vi "find strasse.vi"(11 "Karte in":T1={"Kreuzungen"=[{"Name"="A1", "Identifikation"=0, "Koord"={"x"=100.0, "y"=100.0}, "Anzahl Abgänge"=1}, {"Name"="A2", "Identifikation"=1, "Koord"={"x"=180.0, "y"=180.0}, "Anzahl Abgänge"=1}, {"Name"="A3", "Identifikation"=2, "Koord"={"x"=210.0, "y"=210.0}, "Anzahl Abgänge"=3}, {"Name"="A4", "Identifikation"=3, "Koord"={"x"=300.0, "y"=300.0}, "Anzahl Abgänge"=3}, {"Name"="A5", "Identifikation"=4, "Koord"={"x"=320.0, "y"=320.0}, "Anzahl Abgänge"=1}, {"Name"="A6", "Identifikation"=5, "Koord"={"x"=40.0, "y"=40.0}, "Anzahl Abgänge"=1}, {"Name"="A7", "Identifikation"=6, "Koord"={"x"=90.0, "y"=90.0}, "Anzahl Abgänge"=3}, {"Name"="A8", "Identifikation"=7, "Koord"={"x"=100.0, "y"=100.0}, "Anzahl Abgänge"=2}, {"Name"="A9", "Identifikation"=8, "Koord"={"x"=90.0, "y"=90.0}, "Anzahl Abgänge"=3}, {"Name"="A10", "Identifikation"=9, "Koord"={"x"=180.0, "y"=180.0}, "Anzahl Abgänge"=3}, {"Name"="A11", "Identifikation"=10, "Koord"={"x"=210.0, "y"=210.0}, "Anzahl Abgänge"=3}, {"Name"="A12", "Identifikation"=11, "Koord"={"x"=180.0, "y"=180.0}, "Anzahl Abgänge"=3}, {"Name"="A13", "Identifikation"=12, "Koord"={"x"=210.0, "y"=210.0}, "Anzahl Abgänge"=3}, {"Name"="A14", "Identifikation"=13, "Koord"={"x"=270.0, "y"=270.0}, "Anzahl Abgänge"=3}, {"Name"="A15", "Identifikation"=14, "Koord"={"x"=300.0, "y"=300.0}, "Anzahl Abgänge"=1}, {"Name"="A16", "Identifikation"=15, "Koord"={"x"=270.0, "y"=270.0}, "Anzahl Abgänge"=3}, {"Name"="A17", "Identifikation"=16, "Koord"={"x"=340.0, "y"=340.0}, "Anzahl Abgänge"=1}, {"Name"="A18", "Identifikation"=17, "Koord"={"x"=180.0, "y"=180.0}, "Anzahl Abgänge"=1}, {"Name"="A19", "Identifikation"=18, "Koord"={"x"=90.0, "y"=90.0}, "Anzahl Abgänge"=1}, {"Name"="A20", "Identifikation"=19, "Koord"={"x"=60.0, "y"=60.0}, "Anzahl Abgänge"=2}, {"Name"="A21", "Identifikation"=20, "Koord"={"x"=160.0, "y"=160.0}, "Anzahl Abgänge"=2}, {"Name"="A22", "Identifikation"=21, "Koord"={"x"=60.0, "y"=60.0}, "Anzahl Abgänge"=1}, {"Name"="A23", "Identifikation"=22, "Koord"={"x"=160.0, "y"=160.0}, "Anzahl Abgänge"=2}, {"Name"="A24", "Identifikation"=23, "Koord"={"x"=270.0, "y"=270.0}, "Anzahl Abgänge"=3}, {"Name"="A25", "Identifikation"=24, "Koord"={"x"=340.0, "y"=340.0}, "Anzahl Abgänge"=1}], "Strassen"=[{"Name"="A 1 8", "Identifikation"=0, "Verbindungen"=[{"Start_Kr"=0, "Ziel_Kr"=7}, {"Start_Kr"=7, "Ziel_Kr"=0}], "Breite"=40, "Strassen_Typ"=enum."Stadt"}, {"Name"="A 2 3", "Identifikation"=1, "Verbindungen"=[{"Start_Kr"=1, "Ziel_Kr"=2}, {"Start_Kr"=2, "Ziel_Kr"=1}], "Breite"=40, "Strassen_Typ"=enum."Innenstadt"}, {"Name"="A 3 4", "Identifikation"=2, "Verbindungen"=[{"Start_Kr"=2, "Ziel_Kr"=3}, {"Start_Kr"=3, "Ziel_Kr"=2}], "Breite"=40, "Strassen_Typ"=enum."Innenstadt"}, {"Name"="A 311", "Identifikation"=3, "Verbindungen"=[{"Start_Kr"=2, "Ziel_Kr"=10}, {"Start_Kr"=10, "Ziel_Kr"=2}], "Breite"=40, "Strassen_Typ"=enum."Innenstadt"}, {"Name"="A 4 5", "Identifikation"=4, "Verbindungen"=[{"Start_Kr"=3, "Ziel_Kr"=4}, {"Start_Kr"=4, "Ziel_Kr"=3}], "Breite"=40, "Strassen_Typ"=enum."Innenstadt"}, {"Name"="A 6 7", "Identifikation"=5, "Verbindungen"=[{"Start_Kr"=5, "Ziel_Kr"=6}, {"Start_Kr"=6, "Ziel_Kr"=5}], "Breite"=40, "Strassen_Typ"=enum."Stadt"}, {"Name"="A 7 8", "Identifikation"=6, "Verbindungen"=[{"Start_Kr"=6, "Ziel_Kr"=7}, {"Start_Kr"=7, "Ziel_Kr"=6}], "Breite"=40, "Strassen_Typ"=enum."Stadt"}, {"Name"="A 7 9", "Identifikation"=7, "Verbindungen"=[{"Start_Kr"=6, "Ziel_Kr"=8}, {"Start_Kr"=8, "Ziel_Kr"=6}], "Breite"=40, "Strassen_Typ"=enum."Stadt"}, {"Name"="A 910", "Identifikation"=8, "Verbindungen"=[{"Start_Kr"=8, "Ziel_Kr"=9}, {"Start_Kr"=9, "Ziel_Kr"=8}], "Breite"=40, "Strassen_Typ"=enum."Innenstadt"}, {"Name"="A 919", "Identifikation"=9, "Verbindungen"=[{"Start_Kr"=8, "Ziel_Kr"=18}, {"Start_Kr"=18, "Ziel_Kr"=8}], "Breite"=40, "Strassen_Typ"=enum."Stadt"}, {"Name"="A1011", "Identifikation"=10, "Verbindungen"=[{"Start_Kr"=9, "Ziel_Kr"=10}, {"Start_Kr"=10, "Ziel_Kr"=9}], "Breite"=40, "Strassen_Typ"=enum."Innenstadt"}, {"Name"="A1012", "Identifikation"=11, "Verbindungen"=[{"Start_Kr"=9, "Ziel_Kr"=11}, {"Start_Kr"=11, "Ziel_Kr"=9}], "Breite"=40, "Strassen_Typ"=enum."Innenstadt"}, {"Name"="A1113", "Identifikation"=12, "Verbindungen"=[{"Start_Kr"=10, "Ziel_Kr"=12}, {"Start_Kr"=12, "Ziel_Kr"=10}], "Breite"=40, "Strassen_Typ"=enum."Innenstadt"}, {"Name"="A1213", "Identifikation"=13, "Verbindungen"=[{"Start_Kr"=11, "Ziel_Kr"=12}, {"Start_Kr"=12, "Ziel_Kr"=11}], "Breite"=40, "Strassen_Typ"=enum."Innenstadt"}, {"Name"="A1218", "Identifikation"=14, "Verbindungen"=[{"Start_Kr"=11, "Ziel_Kr"=17}, {"Start_Kr"=17, "Ziel_Kr"=11}], "Breite"=40, "Strassen_Typ"=enum."Innenstadt"}, {"Name"="A1314", "Identifikation"=15, "Verbindungen"=[{"Start_Kr"=12, "Ziel_Kr"=13}, {"Start_Kr"=13, "Ziel_Kr"=12}], "Breite"=40, "Strassen_Typ"=enum."Innenstadt"}, {"Name"="A1415", "Identifikation"=16, "Verbindungen"=[{"Start_Kr"=13, "Ziel_Kr"=14}, {"Start_Kr"=14, "Ziel_Kr"=13}], "Breite"=40, "Strassen_Typ"=enum."Innenstadt"}, {"Name"="A1416", "Identifikation"=17, "Verbindungen"=[{"Start_Kr"=13, "Ziel_Kr"=15}, {"Start_Kr"=15, "Ziel_Kr"=13}], "Breite"=40, "Strassen_Typ"=enum."Innenstadt"}, {"Name"="A 415", "Identifikation"=18, "Verbindungen"=[{"Start_Kr"=14, "Ziel_Kr"=3}], "Breite"=40, "Strassen_Typ"=enum."Innenstadt"}, {"Name"="A1617", "Identifikation"=19, "Verbindungen"=[{"Start_Kr"=15, "Ziel_Kr"=16}, {"Start_Kr"=16, "Ziel_Kr"=15}], "Breite"=40, "Strassen_Typ"=enum."Stadt"}, {"Name"="A1624", "Identifikation"=20, "Verbindungen"=[{"Start_Kr"=15, "Ziel_Kr"=23}, {"Start_Kr"=23, "Ziel_Kr"=15}], "Breite"=40, "Strassen_Typ"=enum."Stadt"}, {"Name"="A2021", "Identifikation"=21, "Verbindungen"=[{"Start_Kr"=19, "Ziel_Kr"=20}, {"Start_Kr"=20, "Ziel_Kr"=19}], "Breite"=40, "Strassen_Typ"=enum."Land"}, {"Name"="A2022", "Identifikation"=22, "Verbindungen"=[{"Start_Kr"=19, "Ziel_Kr"=21}, {"Start_Kr"=21, "Ziel_Kr"=19}], "Breite"=40, "Strassen_Typ"=enum."Land"}, {"Name"="A2123", "Identifikation"=23, "Verbindungen"=[{"Start_Kr"=20, "Ziel_Kr"=22}, {"Start_Kr"=22, "Ziel_Kr"=20}], "Breite"=40, "Strassen_Typ"=enum."Land"}, {"Name"="A2324", "Identifikation"=24, "Verbindungen"=[{"Start_Kr"=22, "Ziel_Kr"=23}, {"Start_Kr"=23, "Ziel_Kr"=22}], "Breite"=40, "Strassen_Typ"=enum."Land"}, {"Name"="A2425", "Identifikation"=25, "Verbindungen"=[{"Start_Kr"=23, "Ziel_Kr"=24}, {"Start_Kr"=24, "Ziel_Kr"=23}], "Breite"=40, "Strassen_Typ"=enum."Land"}], "Häuser"=[{"Name"="Haus1", "Hausnummer"=0, "Polygon"=[{"x"=220.0, "y"=40.0}, {"x"=280.0, "y"=40.0}, {"x"=280.0, "y"=0.0}, {"x"=220.0, "y"=0.0}, {"x"=250.0, "y"=20.0}], "Strassennummer"=0, "Türe"={"x"=250.0, "y"=40.0}}, {"Name"="Haus2", "Hausnummer"=1, "Polygon"=[{"x"=280.0, "y"=40.0}, {"x"=340.0, "y"=40.0}, {"x"=340.0, "y"=0.0}, {"x"=280.0, "y"=0.0}, {"x"=310.0, "y"=20.0}], "Strassennummer"=0, "Türe"={"x"=310.0, "y"=40.0}}, {"Name"="Haus3", "Hausnummer"=2, "Polygon"=[{"x"=20.0, "y"=60.0}, {"x"=80.0, "y"=60.0}, {"x"=80.0, "y"=20.0}, {"x"=20.0, "y"=20.0}, {"x"=50.0, "y"=40.0}], "Strassennummer"=0, "Türe"={"x"=50.0, "y"=60.0}}, {"Name"="Haus4", "Hausnummer"=3, "Polygon"=[{"x"=120.0, "y"=40.0}, {"x"=120.0, "y"=100.0}, {"x"=160.0, "y"=100.0}, {"x"=160.0, "y"=40.0}, {"x"=140.0, "y"=70.0}], "Strassennummer"=0, "Türe"={"x"=120.0, "y"=70.0}}, {"Name"="Haus5", "Hausnummer"=4, "Polygon"=[{"x"=340.0, "y"=40.0}, {"x"=340.0, "y"=100.0}, {"x"=380.0, "y"=100.0}, {"x"=380.0, "y"=40.0}, {"x"=360.0, "y"=70.0}], "Strassennummer"=0, "Türe"={"x"=340.0, "y"=70.0}}, {"Name"="Haus6", "Hausnummer"=5, "Polygon"=[{"x"=20.0, "y"=120.0}, {"x"=20.0, "y"=180.0}, {"x"=60.0, "y"=180.0}, {"x"=60.0, "y"=120.0}, {"x"=40.0, "y"=150.0}], "Strassennummer"=0, "Türe"={"x"=40.0, "y"=120.0}}, {"Name"="Haus7", "Hausnummer"=6, "Polygon"=[{"x"=180.0, "y"=100.0}, {"x"=120.0, "y"=100.0}, {"x"=120.0, "y"=140.0}, {"x"=180.0, "y"=140.0}, {"x"=150.0, "y"=120.0}], "Strassennummer"=0, "Türe"={"x"=180.0, "y"=120.0}}, {"Name"="Haus8", "Hausnummer"=7, "Polygon"=[{"x"=320.0, "y"=140.0}, {"x"=380.0, "y"=140.0}, {"x"=380.0, "y"=100.0}, {"x"=320.0, "y"=100.0}, {"x"=350.0, "y"=120.0}], "Strassennummer"=0, "Türe"={"x"=320.0, "y"=120.0}}, {"Name"="Haus9", "Hausnummer"=8, "Polygon"=[{"x"=240.0, "y"=100.0}, {"x"=240.0, "y"=160.0}, {"x"=280.0, "y"=160.0}, {"x"=280.0, "y"=100.0}, {"x"=260.0, "y"=130.0}], "Strassennummer"=0, "Türe"={"x"=240.0, "y"=130.0}}, {"Name"="Haus10", "Hausnummer"=9, "Polygon"=[{"x"=320.0, "y"=140.0}, {"x"=320.0, "y"=200.0}, {"x"=360.0, "y"=200.0}, {"x"=360.0, "y"=140.0}, {"x"=340.0, "y"=170.0}], "Strassennummer"=0, "Türe"={"x"=320.0, "y"=170.0}}, {"Name"="Haus11", "Hausnummer"=10, "Polygon"=[{"x"=45.0, "y"=240.0}, {"x"=45.0, "y"=180.0}, {"x"=5.0, "y"=180.0}, {"x"=5.0, "y"=240.0}, {"x"=25.0, "y"=210.0}], "Strassennummer"=0, "Türe"={"x"=45.0, "y"=210.0}}, {"Name"="Haus12", "Hausnummer"=11, "Polygon"=[{"x"=200.0, "y"=220.0}, {"x"=200.0, "y"=280.0}, {"x"=240.0, "y"=280.0}, {"x"=240.0, "y"=220.0}, {"x"=220.0, "y"=250.0}], "Strassennummer"=0, "Türe"={"x"=220.0, "y"=220.0}}, {"Name"="Haus13", "Hausnummer"=12, "Polygon"=[{"x"=160.0, "y"=260.0}, {"x"=160.0, "y"=200.0}, {"x"=120.0, "y"=200.0}, {"x"=120.0, "y"=260.0}, {"x"=140.0, "y"=230.0}], "Strassennummer"=0, "Türe"={"x"=160.0, "y"=230.0}}, {"Name"="Haus14", "Hausnummer"=13, "Polygon"=[{"x"=60.0, "y"=240.0}, {"x"=0.0, "y"=240.0}, {"x"=0.0, "y"=280.0}, {"x"=60.0, "y"=280.0}, {"x"=30.0, "y"=260.0}], "Strassennummer"=0, "Türe"={"x"=60.0, "y"=260.0}}, {"Name"="Haus15", "Hausnummer"=14, "Polygon"=[{"x"=360.0, "y"=280.0}, {"x"=300.0, "y"=280.0}, {"x"=300.0, "y"=320.0}, {"x"=360.0, "y"=320.0}, {"x"=330.0, "y"=300.0}], "Strassennummer"=0, "Türe"={"x"=330.0, "y"=280.0}}, {"Name"="Haus16", "Hausnummer"=15, "Polygon"=[{"x"=130.0, "y"=300.0}, {"x"=190.0, "y"=300.0}, {"x"=190.0, "y"=260.0}, {"x"=130.0, "y"=260.0}, {"x"=160.0, "y"=280.0}], "Strassennummer"=0, "Türe"={"x"=160.0, "y"=300.0}}, {"Name"="Haus17", "Hausnummer"=16, "Polygon"=[{"x"=240.0, "y"=350.0}, {"x"=240.0, "y"=290.0}, {"x"=200.0, "y"=290.0}, {"x"=200.0, "y"=350.0}, {"x"=220.0, "y"=320.0}], "Strassennummer"=0, "Türe"={"x"=240.0, "y"=320.0}}, {"Name"="Haus18", "Hausnummer"=17, "Polygon"=[{"x"=300.0, "y"=360.0}, {"x"=360.0, "y"=360.0}, {"x"=360.0, "y"=320.0}, {"x"=300.0, "y"=320.0}, {"x"=330.0, "y"=340.0}], "Strassennummer"=0, "Türe"={"x"=330.0, "y"=360.0}}, {"Name"="Haus19", "Hausnummer"=18, "Polygon"=[{"x"=90.0, "y"=400.0}, {"x"=30.0, "y"=400.0}, {"x"=30.0, "y"=440.0}, {"x"=90.0, "y"=440.0}, {"x"=60.0, "y"=420.0}], "Strassennummer"=0, "Türe"={"x"=60.0, "y"=400.0}}, {"Name"="Poststelle", "Hausnummer"=19, "Polygon"=[{"x"=160.0, "y"=40.0}, {"x"=220.0, "y"=40.0}, {"x"=220.0, "y"=0.0}, {"x"=160.0, "y"=0.0}, {"x"=190.0, "y"=20.0}], "Strassennummer"=0, "Türe"={"x"=190.0, "y"=40.0}}]}) -> (3 "Karte out":T1={"Kreuzungen"=[{"Name"="A1", "Identifikation"=0, "Koord"={"x"=100.0, "y"=100.0}, "Anzahl Abgänge"=1}, {"Name"="A2", "Identifikation"=1, "Koord"={"x"=180.0, "y"=180.0}, "Anzahl Abgänge"=1}, {"Name"="A3", "Identifikation"=2, "Koord"={"x"=210.0, "y"=210.0}, "Anzahl Abgänge"=3}, {"Name"="A4", "Identifikation"=3, "Koord"={"x"=300.0, "y"=300.0}, "Anzahl Abgänge"=3}, {"Name"="A5", "Identifikation"=4, "Koord"={"x"=320.0, "y"=320.0}, "Anzahl Abgänge"=1}, {"Name"="A6", "Identifikation"=5, "Koord"={"x"=40.0, "y"=40.0}, "Anzahl Abgänge"=1}, {"Name"="A7", "Identifikation"=6, "Koord"={"x"=90.0, "y"=90.0}, "Anzahl Abgänge"=3}, {"Name"="A8", "Identifikation"=7, "Koord"={"x"=100.0, "y"=100.0}, "Anzahl Abgänge"=2}, {"Name"="A9", "Identifikation"=8, "Koord"={"x"=90.0, "y"=90.0}, "Anzahl Abgänge"=3}, {"Name"="A10", "Identifikation"=9, "Koord"={"x"=180.0, "y"=180.0}, "Anzahl Abgänge"=3}, {"Name"="A11", "Identifikation"=10, "Koord"={"x"=210.0, "y"=210.0}, "Anzahl Abgänge"=3}, {"Name"="A12", "Identifikation"=11, "Koord"={"x"=180.0, "y"=180.0}, "Anzahl Abgänge"=3}, {"Name"="A13", "Identifikation"=12, "Koord"={"x"=210.0, "y"=210.0}, "Anzahl Abgänge"=3}, {"Name"="A14", "Identifikation"=13, "Koord"={"x"=270.0, "y"=270.0}, "Anzahl Abgänge"=3}, {"Name"="A15", "Identifikation"=14, "Koord"={"x"=300.0, "y"=300.0}, "Anzahl Abgänge"=1}, {"Name"="A16", "Identifikation"=15, "Koord"={"x"=270.0, "y"=270.0}, "Anzahl Abgänge"=3}, {"Name"="A17", "Identifikation"=16, "Koord"={"x"=340.0, "y"=340.0}, "Anzahl Abgänge"=1}, {"Name"="A18", "Identifikation"=17, "Koord"={"x"=180.0, "y"=180.0}, "Anzahl Abgänge"=1}, {"Name"="A19", "Identifikation"=18, "Koord"={"x"=90.0, "y"=90.0}, "Anzahl Abgänge"=1}, {"Name"="A20", "Identifikation"=19, "Koord"={"x"=60.0, "y"=60.0}, "Anzahl Abgänge"=2}, {"Name"="A21", "Identifikation"=20, "Koord"={"x"=160.0, "y"=160.0}, "Anzahl Abgänge"=2}, {"Name"="A22", "Identifikation"=21, "Koord"={"x"=60.0, "y"=60.0}, "Anzahl Abgänge"=1}, {"Name"="A23", "Identifikation"=22, "Koord"={"x"=160.0, "y"=160.0}, "Anzahl Abgänge"=2}, {"Name"="A24", "Identifikation"=23, "Koord"={"x"=270.0, "y"=270.0}, "Anzahl Abgänge"=3}, {"Name"="A25", "Identifikation"=24, "Koord"={"x"=340.0, "y"=340.0}, "Anzahl Abgänge"=1}], "Strassen"=[{"Name"="A 1 8", "Identifikation"=0, "Verbindungen"=[{"Start_Kr"=0, "Ziel_Kr"=7}, {"Start_Kr"=7, "Ziel_Kr"=0}], "Breite"=40, "Strassen_Typ"=enum."Stadt"}, {"Name"="A 2 3", "Identifikation"=1, "Verbindungen"=[{"Start_Kr"=1, "Ziel_Kr"=2}, {"Start_Kr"=2, "Ziel_Kr"=1}], "Breite"=40, "Strassen_Typ"=enum."Innenstadt"}, {"Name"="A 3 4", "Identifikation"=2, "Verbindungen"=[{"Start_Kr"=2, "Ziel_Kr"=3}, {"Start_Kr"=3, "Ziel_Kr"=2}], "Breite"=40, "Strassen_Typ"=enum."Innenstadt"}, {"Name"="A 311", "Identifikation"=3, "Verbindungen"=[{"Start_Kr"=2, "Ziel_Kr"=10}, {"Start_Kr"=10, "Ziel_Kr"=2}], "Breite"=40, "Strassen_Typ"=enum."Innenstadt"}, {"Name"="A 4 5", "Identifikation"=4, "Verbindungen"=[{"Start_Kr"=3, "Ziel_Kr"=4}, {"Start_Kr"=4, "Ziel_Kr"=3}], "Breite"=40, "Strassen_Typ"=enum."Innenstadt"}, {"Name"="A 6 7", "Identifikation"=5, "Verbindungen"=[{"Start_Kr"=5, "Ziel_Kr"=6}, {"Start_Kr"=6, "Ziel_Kr"=5}], "Breite"=40, "Strassen_Typ"=enum."Stadt"}, {"Name"="A 7 8", "Identifikation"=6, "Verbindungen"=[{"Start_Kr"=6, "Ziel_Kr"=7}, {"Start_Kr"=7, "Ziel_Kr"=6}], "Breite"=40, "Strassen_Typ"=enum."Stadt"}, {"Name"="A 7 9", "Identifikation"=7, "Verbindungen"=[{"Start_Kr"=6, "Ziel_Kr"=8}, {"Start_Kr"=8, "Ziel_Kr"=6}], "Breite"=40, "Strassen_Typ"=enum."Stadt"}, {"Name"="A 910", "Identifikation"=8, "Verbindungen"=[{"Start_Kr"=8, "Ziel_Kr"=9}, {"Start_Kr"=9, "Ziel_Kr"=8}], "Breite"=40, "Strassen_Typ"=enum."Innenstadt"}, {"Name"="A 919", "Identifikation"=9, "Verbindungen"=[{"Start_Kr"=8, "Ziel_Kr"=18}, {"Start_Kr"=18, "Ziel_Kr"=8}], "Breite"=40, "Strassen_Typ"=enum."Stadt"}, {"Name"="A1011", "Identifikation"=10, "Verbindungen"=[{"Start_Kr"=9, "Ziel_Kr"=10}, {"Start_Kr"=10, "Ziel_Kr"=9}], "Breite"=40, "Strassen_Typ"=enum."Innenstadt"}, {"Name"="A1012", "Identifikation"=11, "Verbindungen"=[{"Start_Kr"=9, "Ziel_Kr"=11}, {"Start_Kr"=11, "Ziel_Kr"=9}], "Breite"=40, "Strassen_Typ"=enum."Innenstadt"}, {"Name"="A1113", "Identifikation"=12, "Verbindungen"=[{"Start_Kr"=10, "Ziel_Kr"=12}, {"Start_Kr"=12, "Ziel_Kr"=10}], "Breite"=40, "Strassen_Typ"=enum."Innenstadt"}, {"Name"="A1213", "Identifikation"=13, "Verbindungen"=[{"Start_Kr"=11, "Ziel_Kr"=12}, {"Start_Kr"=12, "Ziel_Kr"=11}], "Breite"=40, "Strassen_Typ"=enum."Innenstadt"}, {"Name"="A1218", "Identifikation"=14, "Verbindungen"=[{"Start_Kr"=11, "Ziel_Kr"=17}, {"Start_Kr"=17, "Ziel_Kr"=11}], "Breite"=40, "Strassen_Typ"=enum."Innenstadt"}, {"Name"="A1314", "Identifikation"=15, "Verbindungen"=[{"Start_Kr"=12, "Ziel_Kr"=13}, {"Start_Kr"=13, "Ziel_Kr"=12}], "Breite"=40, "Strassen_Typ"=enum."Innenstadt"}, {"Name"="A1415", "Identifikation"=16, "Verbindungen"=[{"Start_Kr"=13, "Ziel_Kr"=14}, {"Start_Kr"=14, "Ziel_Kr"=13}], "Breite"=40, "Strassen_Typ"=enum."Innenstadt"}, {"Name"="A1416", "Identifikation"=17, "Verbindungen"=[{"Start_Kr"=13, "Ziel_Kr"=15}, {"Start_Kr"=15, "Ziel_Kr"=13}], "Breite"=40, "Strassen_Typ"=enum."Innenstadt"}, {"Name"="A 415", "Identifikation"=18, "Verbindungen"=[{"Start_Kr"=14, "Ziel_Kr"=3}], "Breite"=40, "Strassen_Typ"=enum."Innenstadt"}, {"Name"="A1617", "Identifikation"=19, "Verbindungen"=[{"Start_Kr"=15, "Ziel_Kr"=16}, {"Start_Kr"=16, "Ziel_Kr"=15}], "Breite"=40, "Strassen_Typ"=enum."Stadt"}, {"Name"="A1624", "Identifikation"=20, "Verbindungen"=[{"Start_Kr"=15, "Ziel_Kr"=23}, {"Start_Kr"=23, "Ziel_Kr"=15}], "Breite"=40, "Strassen_Typ"=enum."Stadt"}, {"Name"="A2021", "Identifikation"=21, "Verbindungen"=[{"Start_Kr"=19, "Ziel_Kr"=20}, {"Start_Kr"=20, "Ziel_Kr"=19}], "Breite"=40, "Strassen_Typ"=enum."Land"}, {"Name"="A2022", "Identifikation"=22, "Verbindungen"=[{"Start_Kr"=19, "Ziel_Kr"=21}, {"Start_Kr"=21, "Ziel_Kr"=19}], "Breite"=40, "Strassen_Typ"=enum."Land"}, {"Name"="A2123", "Identifikation"=23, "Verbindungen"=[{"Start_Kr"=20, "Ziel_Kr"=22}, {"Start_Kr"=22, "Ziel_Kr"=20}], "Breite"=40, "Strassen_Typ"=enum."Land"}, {"Name"="A2324", "Identifikation"=24, "Verbindungen"=[{"Start_Kr"=22, "Ziel_Kr"=23}, {"Start_Kr"=23, "Ziel_Kr"=22}], "Breite"=40, "Strassen_Typ"=enum."Land"}, {"Name"="A2425", "Identifikation"=25, "Verbindungen"=[{"Start_Kr"=23, "Ziel_Kr"=24}, {"Start_Kr"=24, "Ziel_Kr"=23}], "Breite"=40, "Strassen_Typ"=enum."Land"}], "Häuser"=[{"Name"="Haus1", "Hausnummer"=0, "Polygon"=[{"x"=220.0, "y"=40.0}, {"x"=280.0, "y"=40.0}, {"x"=280.0, "y"=0.0}, {"x"=220.0, "y"=0.0}, {"x"=250.0, "y"=20.0}], "Strassennummer"=21, "Türe"={"x"=250.0, "y"=40.0}}, {"Name"="Haus2", "Hausnummer"=1, "Polygon"=[{"x"=280.0, "y"=40.0}, {"x"=340.0, "y"=40.0}, {"x"=340.0, "y"=0.0}, {"x"=280.0, "y"=0.0}, {"x"=310.0, "y"=20.0}], "Strassennummer"=24, "Türe"={"x"=310.0, "y"=40.0}}, {"Name"="Haus3", "Hausnummer"=2, "Polygon"=[{"x"=20.0, "y"=60.0}, {"x"=80.0, "y"=60.0}, {"x"=80.0, "y"=20.0}, {"x"=20.0, "y"=20.0}, {"x"=50.0, "y"=40.0}], "Strassennummer"=21, "Türe"={"x"=50.0, "y"=60.0}}, {"Name"="Haus4", "Hausnummer"=3, "Polygon"=[{"x"=120.0, "y"=40.0}, {"x"=120.0, "y"=100.0}, {"x"=160.0, "y"=100.0}, {"x"=160.0, "y"=40.0}, {"x"=140.0, "y"=70.0}], "Strassennummer"=21, "Türe"={"x"=120.0, "y"=70.0}}, {"Name"="Haus5", "Hausnummer"=4, "Polygon"=[{"x"=340.0, "y"=40.0}, {"x"=340.0, "y"=100.0}, {"x"=380.0, "y"=100.0}, {"x"=380.0, "y"=40.0}, {"x"=360.0, "y"=70.0}], "Strassennummer"=24, "Türe"={"x"=340.0, "y"=70.0}}, {"Name"="Haus6", "Hausnummer"=5, "Polygon"=[{"x"=20.0, "y"=120.0}, {"x"=20.0, "y"=180.0}, {"x"=60.0, "y"=180.0}, {"x"=60.0, "y"=120.0}, {"x"=40.0, "y"=150.0}], "Strassennummer"=0, "Türe"={"x"=40.0, "y"=120.0}}, {"Name"="Haus7", "Hausnummer"=6, "Polygon"=[{"x"=180.0, "y"=100.0}, {"x"=120.0, "y"=100.0}, {"x"=120.0, "y"=140.0}, {"x"=180.0, "y"=140.0}, {"x"=150.0, "y"=120.0}], "Strassennummer"=8, "Türe"={"x"=180.0, "y"=120.0}}, {"Name"="Haus8", "Hausnummer"=7, "Polygon"=[{"x"=320.0, "y"=140.0}, {"x"=380.0, "y"=140.0}, {"x"=380.0, "y"=100.0}, {"x"=320.0, "y"=100.0}, {"x"=350.0, "y"=120.0}], "Strassennummer"=24, "Türe"={"x"=320.0, "y"=120.0}}, {"Name"="Haus9", "Hausnummer"=8, "Polygon"=[{"x"=240.0, "y"=100.0}, {"x"=240.0, "y"=160.0}, {"x"=280.0, "y"=160.0}, {"x"=280.0, "y"=100.0}, {"x"=260.0, "y"=130.0}], "Strassennummer"=24, "Türe"={"x"=240.0, "y"=130.0}}, {"Name"="Haus10", "Hausnummer"=9, "Polygon"=[{"x"=320.0, "y"=140.0}, {"x"=320.0, "y"=200.0}, {"x"=360.0, "y"=200.0}, {"x"=360.0, "y"=140.0}, {"x"=340.0, "y"=170.0}], "Strassennummer"=2, "Türe"={"x"=320.0, "y"=170.0}}, {"Name"="Haus11", "Hausnummer"=10, "Polygon"=[{"x"=45.0, "y"=240.0}, {"x"=45.0, "y"=180.0}, {"x"=5.0, "y"=180.0}, {"x"=5.0, "y"=240.0}, {"x"=25.0, "y"=210.0}], "Strassennummer"=0, "Türe"={"x"=45.0, "y"=210.0}}, {"Name"="Haus12", "Hausnummer"=11, "Polygon"=[{"x"=200.0, "y"=220.0}, {"x"=200.0, "y"=280.0}, {"x"=240.0, "y"=280.0}, {"x"=240.0, "y"=220.0}, {"x"=220.0, "y"=250.0}], "Strassennummer"=2, "Türe"={"x"=220.0, "y"=220.0}}, {"Name"="Haus13", "Hausnummer"=12, "Polygon"=[{"x"=160.0, "y"=260.0}, {"x"=160.0, "y"=200.0}, {"x"=120.0, "y"=200.0}, {"x"=120.0, "y"=260.0}, {"x"=140.0, "y"=230.0}], "Strassennummer"=1, "Türe"={"x"=160.0, "y"=230.0}}, {"Name"="Haus14", "Hausnummer"=13, "Polygon"=[{"x"=60.0, "y"=240.0}, {"x"=0.0, "y"=240.0}, {"x"=0.0, "y"=280.0}, {"x"=60.0, "y"=280.0}, {"x"=30.0, "y"=260.0}], "Strassennummer"=0, "Türe"={"x"=60.0, "y"=260.0}}, {"Name"="Haus15", "Hausnummer"=14, "Polygon"=[{"x"=360.0, "y"=280.0}, {"x"=300.0, "y"=280.0}, {"x"=300.0, "y"=320.0}, {"x"=360.0, "y"=320.0}, {"x"=330.0, "y"=300.0}], "Strassennummer"=19, "Türe"={"x"=330.0, "y"=280.0}}, {"Name"="Haus16", "Hausnummer"=15, "Polygon"=[{"x"=130.0, "y"=300.0}, {"x"=190.0, "y"=300.0}, {"x"=190.0, "y"=260.0}, {"x"=130.0, "y"=260.0}, {"x"=160.0, "y"=280.0}], "Strassennummer"=1, "Türe"={"x"=160.0, "y"=300.0}}, {"Name"="Haus17", "Hausnummer"=16, "Polygon"=[{"x"=240.0, "y"=350.0}, {"x"=240.0, "y"=290.0}, {"x"=200.0, "y"=290.0}, {"x"=200.0, "y"=350.0}, {"x"=220.0, "y"=320.0}], "Strassennummer"=4, "Türe"={"x"=240.0, "y"=320.0}}, {"Name"="Haus18", "Hausnummer"=17, "Polygon"=[{"x"=300.0, "y"=360.0}, {"x"=360.0, "y"=360.0}, {"x"=360.0, "y"=320.0}, {"x"=300.0, "y"=320.0}, {"x"=330.0, "y"=340.0}], "Strassennummer"=4, "Türe"={"x"=330.0, "y"=360.0}}, {"Name"="Haus19", "Hausnummer"=18, "Polygon"=[{"x"=90.0, "y"=400.0}, {"x"=30.0, "y"=400.0}, {"x"=30.0, "y"=440.0}, {"x"=90.0, "y"=440.0}, {"x"=60.0, "y"=420.0}], "Strassennummer"=0, "Türe"={"x"=60.0, "y"=400.0}}, {"Name"="Poststelle", "Hausnummer"=19, "Polygon"=[{"x"=160.0, "y"=40.0}, {"x"=220.0, "y"=40.0}, {"x"=220.0, "y"=0.0}, {"x"=160.0, "y"=0.0}, {"x"=190.0, "y"=20.0}], "Strassennummer"=21, "Türe"={"x"=190.0, "y"=40.0}}]})   [LabVIEW 2019]
uses:
  Karte.ctl
  Kreuzung.ctl
  Koordinate.ctl
  Strasse.ctl
  Verbindung.ctl
  Strassentyp.ctl
  Haus.ctl
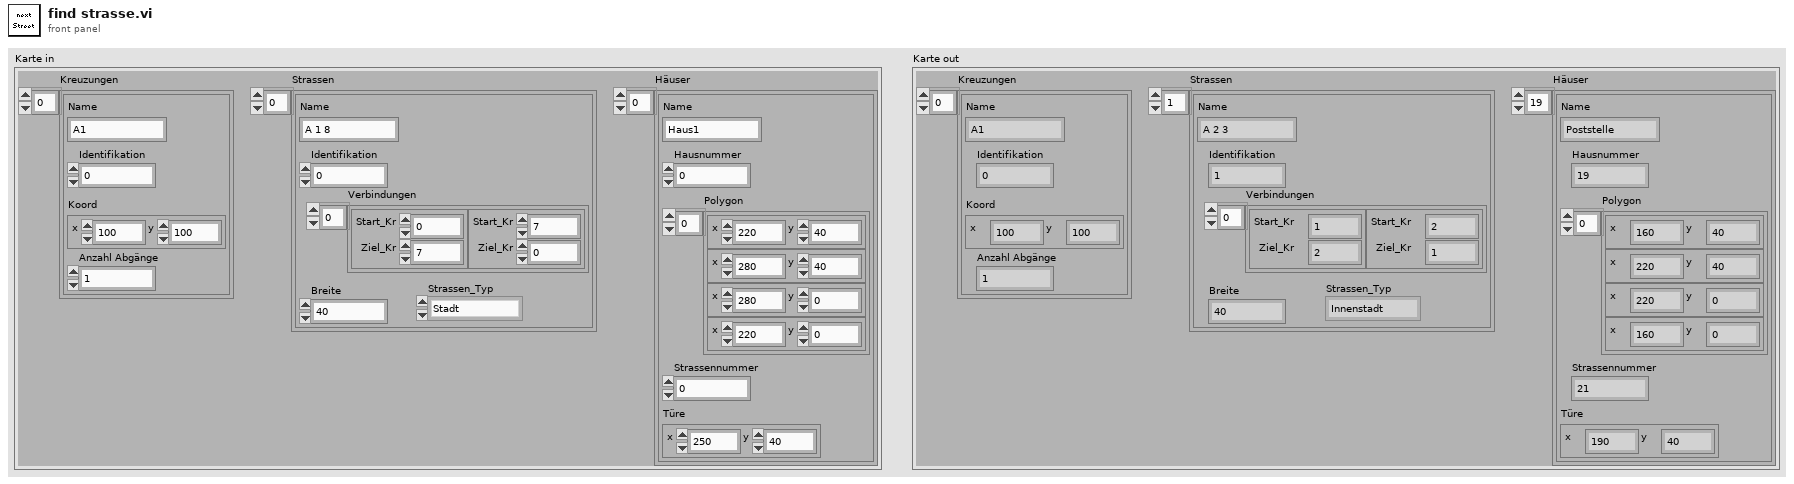
[diagram p1: front panel]
types:
  T1 = typedef "Karte.ctl" = cluster{"Kreuzungen":T2[], "Strassen":T4[], "Häuser":T7[]}
  T2 = typedef "Kreuzung.ctl" = cluster{"Name":string, "Identifikation":u8, "Koord":T3, "Anzahl Abgänge":u8}
  T3 = typedef "Koordinate.ctl" = cluster{"x":dbl, "y":dbl}
  T4 = typedef "Strasse.ctl" = cluster{"Name":string, "Identifikation":u8, "Verbindungen":T5[], "Breite":u8, "Strassen_Typ":T6}
  T5 = typedef "Verbindung.ctl" = cluster{"Start_Kr":u16, "Ziel_Kr":u16}
  T6 = typedef "Strassentyp.ctl" = enum16{"Innenstadt", "Stadt", "Land"}
  T7 = typedef "Haus.ctl" = cluster{"Name":string, "Hausnummer":u8, "Polygon":T3[], "Strassennummer":u8, "Türe":T3}
  T8 = typedef "2_Pt_Strasse.ctl" = cluster{"P1":T3, "P2":T3, "horizontal":bool}
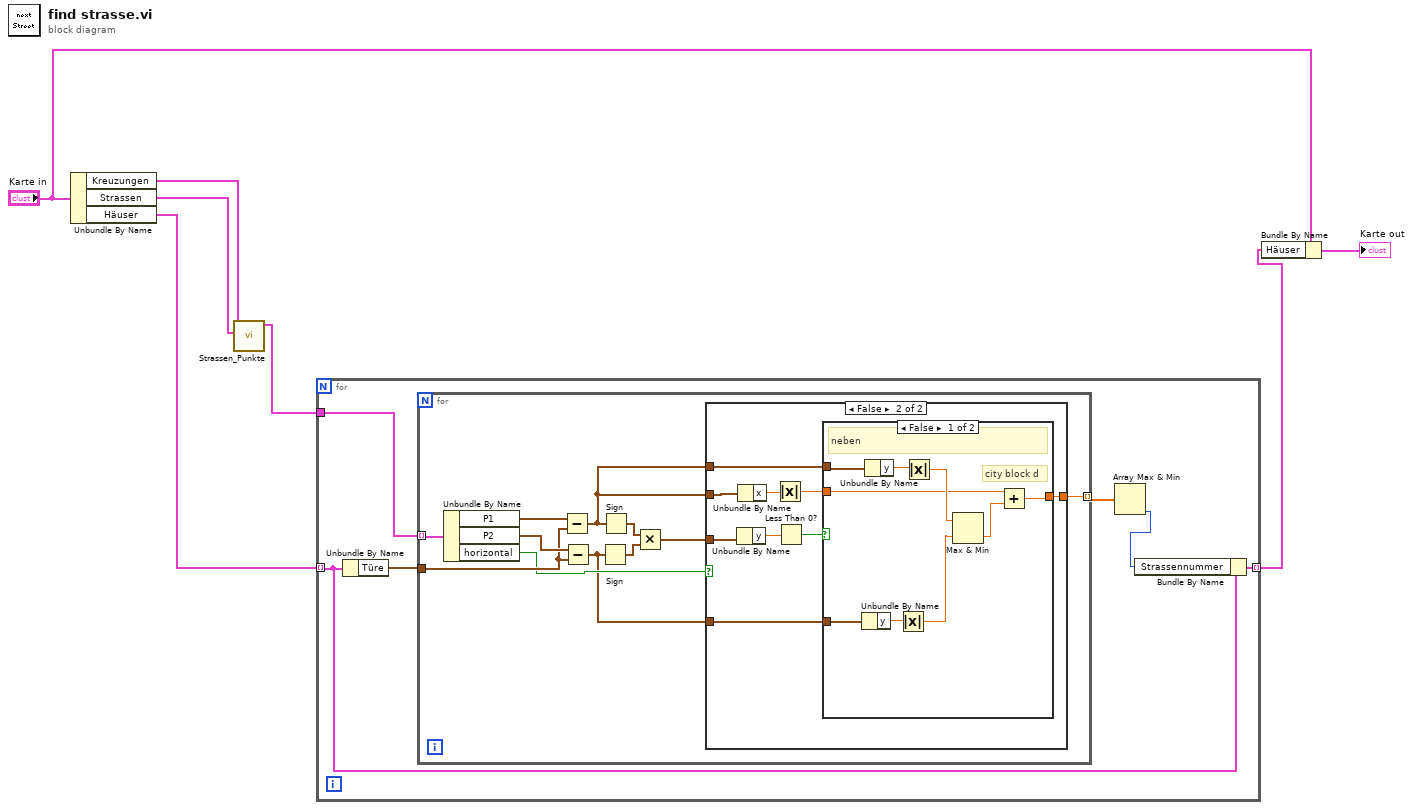
[diagram p0: block diagram]
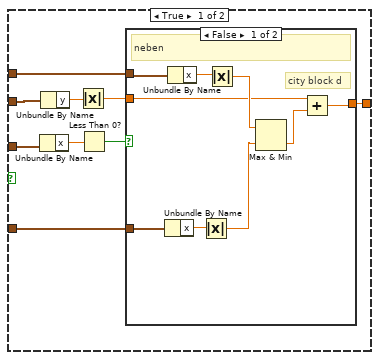
[diagram p2: hidden frame]
diagram:
  n1 = Unbundle By Name("Karte in") -> ("Kreuzungen"=w6:T2[], "Strassen"=w7:T4[], "Häuser"=w5:T7[])
  n2 = call "Strassen_Punkte.vi"("Strassen"=w7, "Kreuzungen"=w6) -> ("Strassenpunkte"=w4:T8[])  [unwired: 9 in]
  n3 = for {
    tunnel: w4 -> [w12]
    tunnel: w5 -> [w10] mode=indexing
    tunnel: [w8] -> w2 mode=indexing
    n4 = Unbundle By Name(w10) -> ("Türe"=w13:T3)
    n5 = for {
      tunnel: w13 -> [w21]
      tunnel: w12 -> [w24] mode=indexing
      tunnel: [w15] -> w11 mode=indexing
      n6 = Unbundle By Name(w24) -> ("P1"=w23:T3, "P2"=w22:T3, "horizontal"=w20:bool)
      n7 = Subtract(x=w23, y=w21) -> (x-y=w14:T3)
      n8 = Subtract(x=w22, y=w21) -> (x-y=w16:T3)
      n9 = Sign(1:w16) -> (0:w18:T3)
      n10 = Sign(1:w14) -> (0:w19:T3)
      n11 = Multiply(x=w19, y=w18) -> (x*y=w17:T3)
      n12 = case shown="False" w20 {
        tunnel: w17 -> [w33 w52]
        tunnel: w16 -> [w30 w49]
        tunnel: w14 -> [w29 w48]
        tunnel: [w27 w46] -> w15
        tunnel: w14 -> [w25 w44]
        frame True {
          n13 = Unbundle By Name(w33) -> ("x"=w32:dbl)
          n14 = Unbundle By Name(w29) -> ("y"=w28:dbl)
          n15 = Absolute Value(x=w28) -> (abs(x)=w26:dbl)
          n16 = Less Than 0?(x=w32) -> (x < 0?=w31:bool)
          n17 = case shown="False" w31 {
            tunnel: w30 -> [w41 _]
            tunnel: [w34 w43] -> w27
            tunnel: w26 -> [w36 w43]
            tunnel: w25 -> [w42 _]
            frame False {
              # "city block d"
              # "neben"
              n18 = Unbundle By Name(w41) -> ("x"=w39:dbl)
              n19 = Unbundle By Name(w42) -> ("x"=w40:dbl)
              n20 = Absolute Value(x=w39) -> (abs(x)=w37:dbl)
              n21 = Absolute Value(x=w40) -> (abs(x)=w38:dbl)
              n22 = Max & Min(x=w38, y=w37) -> (min(x,y)=w35:dbl)  [unwired: 1 out]
              n23 = Add(x=w36, y=w35) -> (x+y=w34:dbl)
            }
            frame True {
              # "Punkt dazwischen"
            }
          }
        }
        frame False {
          n24 = Unbundle By Name(w52) -> ("y"=w51:dbl)
          n25 = Unbundle By Name(w48) -> ("x"=w47:dbl)
          n26 = Absolute Value(x=w47) -> (abs(x)=w45:dbl)
          n27 = Less Than 0?(x=w51) -> (x < 0?=w50:bool)
          n28 = case shown="False" w50 {
            tunnel: w49 -> [w60 _]
            tunnel: [w53 w62] -> w46
            tunnel: w45 -> [w55 w62]
            tunnel: w44 -> [w61 _]
            frame False {
              # "city block d"
              # "neben"
              n29 = Unbundle By Name(w60) -> ("y"=w58:dbl)
              n30 = Unbundle By Name(w61) -> ("y"=w59:dbl)
              n31 = Absolute Value(x=w58) -> (abs(x)=w56:dbl)
              n32 = Absolute Value(x=w59) -> (abs(x)=w57:dbl)
              n33 = Max & Min(x=w57, y=w56) -> (min(x,y)=w54:dbl)  [unwired: 1 out]
              n34 = Add(x=w55, y=w54) -> (x+y=w53:dbl)
            }
            frame True {
              # "Punkt dazwischen"
            }
          }
        }
      }
    }
    n35 = Array Max & Min(array=w11) -> (min index (indices)=w9:i32)  [unwired: 3 out]
    n36 = Bundle By Name(cluster=w10, "Strassennummer"=w9) -> (w8:T7)
  }
  n37 = Bundle By Name(cluster="Karte in", "Häuser"=w2) -> (→"Karte out":T1)
